vi "midi_NoteInfo.vi"(8 "fs [Hz]":dbl, 11 "note event":dbl[](array[numeric])) -> (2 "note info":T1)   [LabVIEW 2013]
doc: "Read note event and return information needed to render audio."
uses:
  midi_NoteInfo.ctl
panel:
  # "midi_NoteInfo"
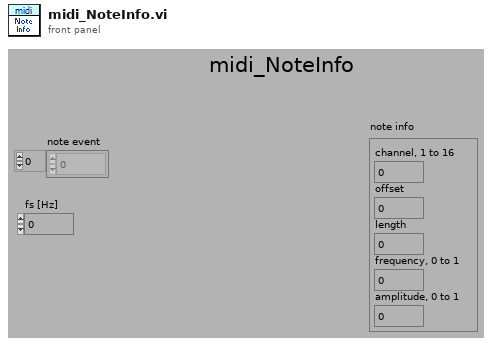
[diagram p1: front panel]
types:
  T1 = typedef "midi_NoteInfo.ctl" = cluster{"channel, 1 to 16":i32, "offset":i32, "length":i32, "frequency, 0 to 1":dbl, "amplitude, 0 to 1":dbl}
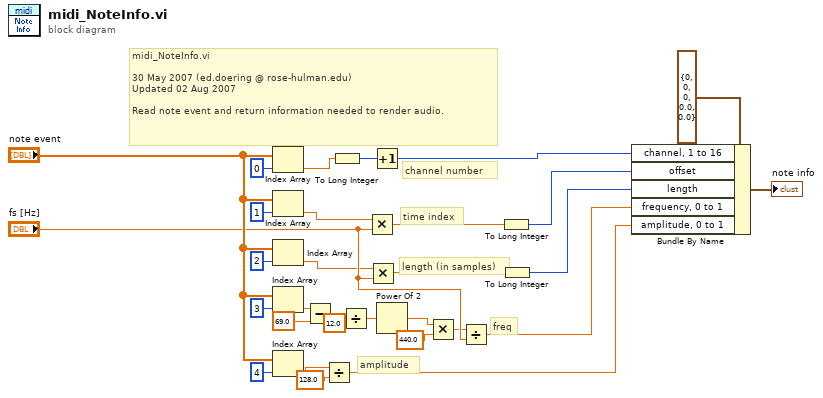
[diagram p0: block diagram]
diagram:
  # "midi_NoteInfo.vi\n\n30 May 2007 (ed.doering @ rose-hulman.edu)\nUpdated 02 Aug 2007\n\nRead note event and return information needed to render audio."
  # "channel number"
  # "amplitude"
  # "freq"
  # "length (in samples)"
  # "time index"
  n1 = Index Array(array="note event", index=0) -> (element=w11:dbl)
  n2 = Index Array(array="note event", index=1) -> (element=w16:dbl)
  n3 = Index Array(array="note event", index=2) -> (element=w15:dbl)
  n4 = Index Array(array="note event", index=3) -> (element=w14:dbl)
  n5 = Index Array(array="note event", index=4) -> (element=w13:dbl)
  n6 = Subtract(x=w14, y=69.0) -> (x-y=w24:dbl)
  n7 = Divide(x=w13, y=128.0) -> (x/y=w1:dbl)
  n8 = To Long Integer(number=w11) -> (32bit integer=w10:i32)
  n9 = Divide(x=w24, y=12.0) -> (x/y=w22:dbl)
  n10 = Multiply(x=w16, y="fs [Hz]") -> (x*y=w9:dbl)
  n11 = Multiply(x=w15, y="fs [Hz]") -> (x*y=w8:dbl)
  n12 = Increment(x=w10) -> (x+1=w5:i32)
  n13 = Power Of 2(x=w22) -> (2^x=w21:dbl)
  n14 = Multiply(x=w21, y=440.0) -> (x*y=w19:dbl)
  n15 = Divide(x=w19, y="fs [Hz]") -> (x/y=w2:dbl)
  n16 = To Long Integer(number=w9) -> (32bit integer=w4:i32)
  n17 = To Long Integer(number=w8) -> (32bit integer=w3:i32)
  n18 = Bundle By Name(cluster=T1 {"channel, 1 to 16"=0, "offset"=0, "length"=0, "frequency, 0 to 1"=0.0, "amplitude, 0 to 1"=0.0} ("note info 2"), "channel, 1 to 16"=w5, "offset"=w4, "length"=w3, "frequency, 0 to 1"=w2, "amplitude, 0 to 1"=w1) -> (→"note info":T1)
